vi "Day 1.vi"() -> ()   [LabVIEW 2020]
uses:
  <vilib>/Utility/file.llb/Read Delimited Spreadsheet (I64).vi
panel:
  out "product":i64
  out "sum":i64
  out "Array":i64[](array[numeric])
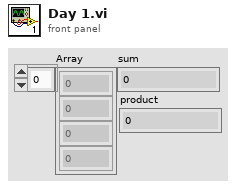
[diagram p1: front panel]
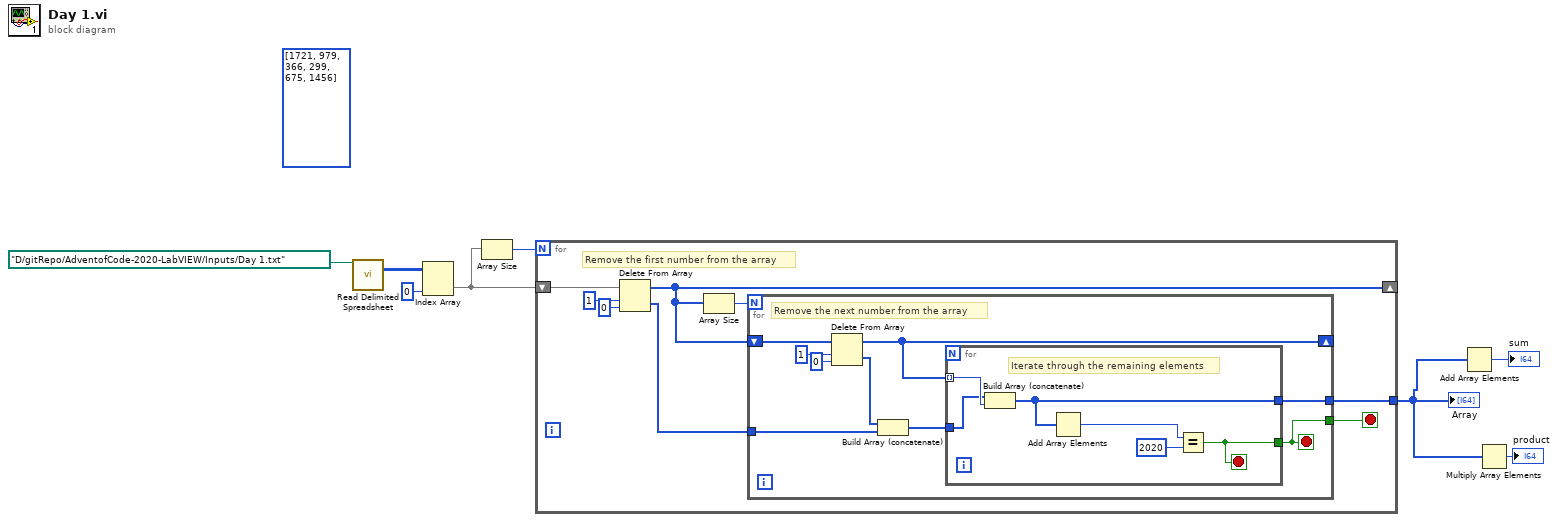
[diagram p0: block diagram]
diagram:
  (unwired) i32[] [1721, 979, 366, 299, 675, 1456]
  n1 = call-poly <vilib>:"Read Delimited Spreadsheet.vi"("file path (dialog if empty)"=path "D:/gitRepo/AdventofCode-2020-LabVIEW/Inputs/Day 1.txt" ("Path")) -> ("all rows"=w6:i64[][])  [unwired: 9 in, 5 out]
  n2 = Index Array(array=w6, index (col)=0 ("disabled index (col)")) -> (element=w4:i64[])  [unwired: 1 in]
  n3 = Array Size(array=w4) -> (size(s)=w8:i32)
  n4 = for {
    N: w8 -> [_]
    shift-right: [w11] -> _
    shift-left: w4 -> [w16]
    tunnel: [w12] -> w2
    stop <- w9 stop-if-true
    # "Remove the first number from the array"
    n5 = Delete From Array(array=w16, length=1, index=0) -> (deleted portion=w13:i64[], array with subset deleted=w11:i64[])
    n6 = Array Size(array=w11) -> (size(s)=w10:i32)
    n7 = for {
      N: w10 -> [_]
      shift-right: [w22] -> _
      shift-left: w11 -> [w25]
      tunnel: w13 -> [w20]
      tunnel: [w18] -> w12
      tunnel: [w17] -> w9
      stop <- w17 stop-if-true
      # "Remove the next number from the array"
      n8 = Delete From Array(array=w25, length=1, index=0) -> (deleted portion=w21:i64[], array with subset deleted=w22:i64[])
      n9 = Build Array (concatenate)(w21, w20) -> (w19:i64[])
      n10 = for {
        tunnel: w22 -> [w29] mode=indexing
        tunnel: w19 -> [w28]
        tunnel: [w30] -> w17
        tunnel: [w26] -> w18
        stop <- w30 stop-if-true
        # "Iterate through the remaining elements"
        n11 = Build Array (concatenate)(w28, w29) -> (w26:i64[])
        n12 = Add Array Elements(numeric array=w26) -> (sum=w27:i64)
        n13 = Equal?(x=w27, y=2020) -> (x = y?=w30:bool)
      }
    }
  }
  "Array" <- w2
  n14 = Add Array Elements(numeric array=w2) -> (sum=→"sum":i64)
  n15 = Multiply Array Elements(1:w2) -> (0:→"product":i64)
